vi "sendHeartbeat.vi"(8 "error in (no error)":errorcluster, 11 "DataListenerThisComponent in":refnum<class "DataListenerThisComponent.lvclass">) -> (0 "error out":errorcluster, 3 "DataListenerThisComponent out":refnum<class "DataListenerThisComponent.lvclass">)   [LabVIEW 2016, in "DataListenerThisComponent.lvclass"]
doc: "Writes heartbeat to shared variable."
uses:
  DataListenerThisComponent.lvclass
  PubSubDataEvent/PubSubDataEvent.lvclass
  ts_sallv_FiberSpectrograph/DataTypes/logevent_heartbeat.ctl
  ts_sallv_FiberSpectrograph/SALLV_FiberSpectrograph.lvlib
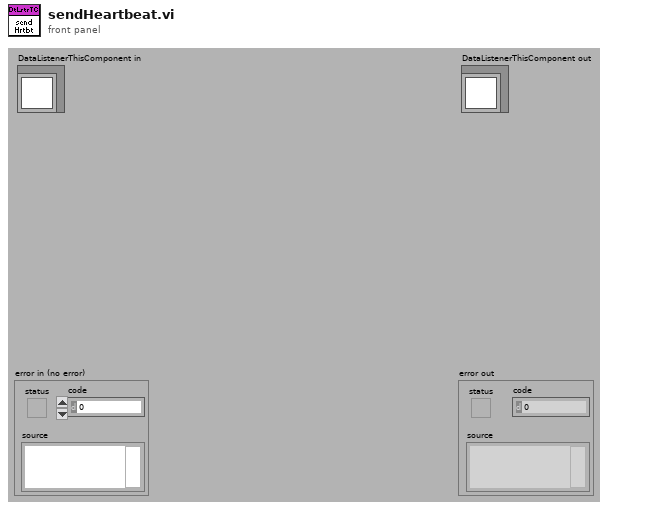
[diagram p1: front panel]
types:
  T1 = typedef "SALLV_FiberSpectrograph.lvlib/logevent_heartbeat.ctl" = cluster{"heartbeat":bool, "priority":i32}
  T2 = typedef "TypedefsDataEvents.lvlib/SubDataEvents.ctl" = cluster{"disable":refnum<user-event>, "enable":refnum<user-event>, "exitControl":refnum<user-event>, "standby":refnum<user-event>, "heartbeat":refnum<user-event>, "start":refnum<user-event>, "captureSpectImage":refnum<user-event>}
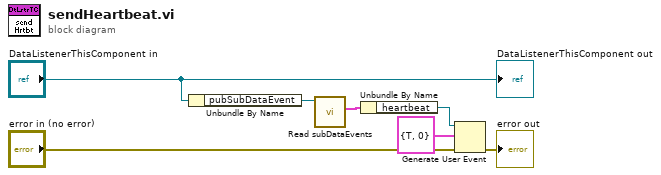
[diagram p0: block diagram]
diagram:
  n1 = Unbundle By Name("DataListenerThisComponent in") -> ("pubSubDataEvent"=w3:refnum<class "PubSubDataEvent.lvclass">)
  n2 = call "Read subDataEvents.vi"("PubSubDataEvent in"=w3) -> ("subDataEvents"=w2:T2)  [unwired: 9 in, 1 out]
  n3 = Unbundle By Name(w2) -> ("heartbeat"=w6:refnum<user-event>)
  n4 = Generate User Event(user event=w6, event data cluster=T1 {"heartbeat"=TRUE, "priority"=0} ("event data"), error in="error in (no error)") -> (error out=→"error out":errorcluster)  [unwired: 1 in, 1 out]
  "DataListenerThisComponent out" <- "DataListenerThisComponent in"
